vi "encoders.vi"   [LabVIEW 2012]
uses:
  Robot Global Data.vi
types:
  T1 = typedef "WPI_EncoderDevRef.ctl" = cluster{"DevStatus":errorcluster, "EncoderIndex":T2, "CounterIndex":T3, "DistancePerCount":dbl, "Decoding Type":T4}
  T2 = typedef "FPGA_EncoderIdx.ctl" = enum8{"Enc 0", "Enc 1", "Enc 2", "Enc 3", "Invalid"}
  T3 = typedef "FPGA_CounterCtrSystemIndex.ctl" = enum8{"Ctr 0", "Ctr 1", "Ctr 2", "Ctr 3", "Ctr 4", "Ctr 5", "Ctr 6", "Ctr 7", "Invalid"}
  T4 = typedef "WPI_EncoderType.ctl" = enum16{"1x", "2x", "4x"}
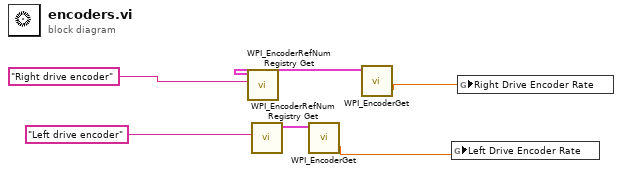
[diagram p0: block diagram]
diagram:
  n1 = call <vilib>:"WPI_EncoderRefNum Registry Get.vi"("refnum name"="Right drive encoder") -> ("EncoderDevRef"=w5:T1)  [unwired: 9 in, 1 out]
  n2 = call <vilib>:"WPI_EncoderRefNum Registry Get.vi"("refnum name"="Left drive encoder") -> ("EncoderDevRef"=w3:T1)  [unwired: 9 in, 1 out]
  n3 = call <vilib>:"WPI_EncoderGet.vi"("EncoderDevRef"=w3) -> ("Rate"=w1:dbl)  [unwired: 5 in, 5 out]
  n4 = call <vilib>:"WPI_EncoderGet.vi"("EncoderDevRef"=w5) -> ("Rate"=w2:dbl)  [unwired: 5 in, 5 out]
  n5 = global write "Robot Global Data.vi" "Left Drive Encoder Rate"(w1) -> ()
  n6 = global write "Robot Global Data.vi" "Right Drive Encoder Rate"(w2) -> ()
